vi "ImageSubset2RPhiArray (SubVI).vi"(8 "error in (no error)":errorcluster, 10 "Fitted Circle":T2, 11 "Full Image in":T1) -> (0 "error out":errorcluster, 1 "2D Array: r, phi, intensity":dbl[][](array[numeric]), 2 "Radius (Pixels)":dbl, 3 "Subset image out":T1)   [LabVIEW 2016]
uses:
  <vilib>/vision/Image Controls.llb/IMAQ Image.ctl
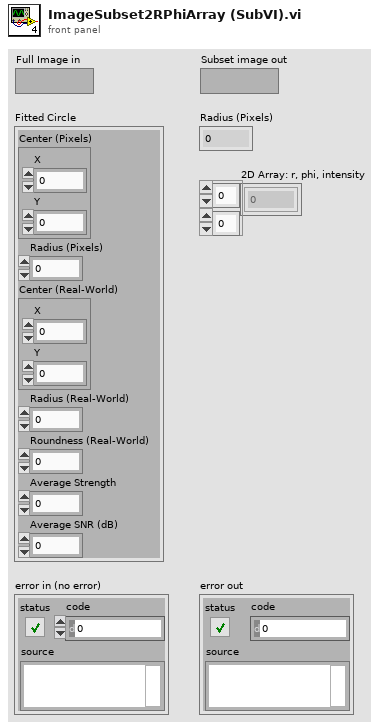
[diagram p1: front panel]
types:
  T1 = typedef "IMAQ Image.ctl" = refnum<image>
  T2 = cluster{"Center (Pixels)":cluster{"X":sgl, "Y":sgl}, "Radius (Pixels)":dbl, "Center (Real-World)":cluster{"X":sgl, "Y":sgl}, "Radius (Real-World)":dbl, "Roundness (Real-World)":dbl, "Average Strength":dbl, "Average SNR (dB)":dbl}
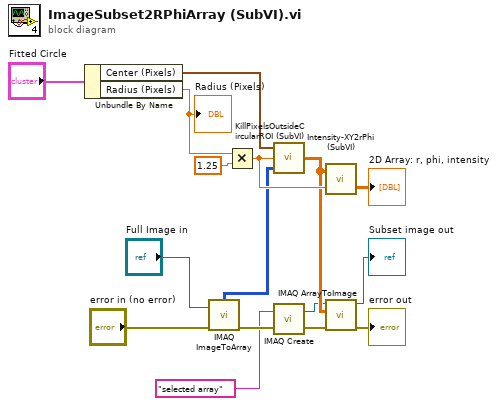
[diagram p0: block diagram]
diagram:
  n1 = Unbundle By Name("Fitted Circle") -> ("Center (Pixels)"=w5:cluster{"X":sgl, "Y":sgl}, "Radius (Pixels)"=w11:dbl)
  "Radius (Pixels)" <- w11
  n2 = call "IMAQ ImageToArray"("error in (no error)"="error in (no error)", "Image"="Full Image in") -> ("error out"=w14:errorcluster, "Image Pixels (U8)"=w4:u8[][])  [unwired: 2 in, 3 out]
  n3 = Multiply(x=w11, y=1.25) -> (x*y=w10:dbl)
  n4 = call "KillPixelsOutsideCircularROI (SubVI).vi"("XY Array"=w4, "Radius*ScaleFactor"=w10, "Center (Pixels)"=w5) -> ("subarray"=w8:dbl[][])
  n5 = call "IMAQ Create"("Image Name"="selected array", "error in (no error)"=w14) -> ("New Image"=w7:T1, "error out"=w15:errorcluster)  [unwired: 3 in]
  n6 = call "Intensity-XY2rPhi (SubVI).vi"("Radius*Scale Factor"=w10, "XY Array"=w8) -> ("2D Array: r, phi, intensity"=→"2D Array: r, phi, intensity":dbl[][])  [unwired: 1 out]
  n7 = call "IMAQ ArrayToImage"("error in (no error)"=w15, "Image Pixels (U8)"=w8, "Image"=w7) -> ("error out"=→"error out":errorcluster, "Image Out"=→"Subset image out":T1)  [unwired: 7 in]
